vi "openCamera.vi"(0 "error in":errorcluster, 2 "Camera Settings":T2={"Camera"=enum."left_hand_camera", "FPS"=20.0, "Camera Controls"=[{"id"=0, "value"=0}, {"id"=101, "value"=-1}, {"id"=102, "value"=-1}, {"id"=103, "value"=-1}, {"id"=104, "value"=-1}, {"id"=105, "value"=-1}, {"id"=106, "value"=-1}, {"id"=107, "value"=-1}, {"id"=108, "value"=-1}, {"id"=109, "value"=1}], "Resolution"=enum."(320, 200)"}, 3 "node":string) -> (1 "error out":errorcluster)   [LabVIEW 2012]
doc: "Opens a connection to a Baxter Camera"
uses:
  ROS/Code/SubVIs/_ROSDirection.ctl
  ROS/Code/Console/Servers/ServerSubs/TopicDef.ctl
  ROS/Code/SubVIs/BaxterCamera.ctl
panel:
  out "Reply":string
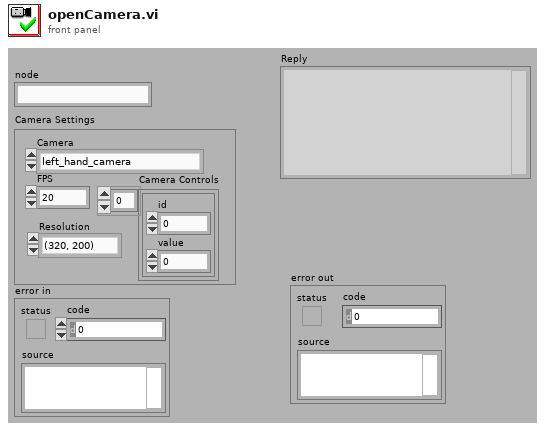
[diagram p1: front panel]
types:
  T1 = typedef "BaxterCamera.ctl" = enum16{"left_hand_camera", "right_hand_camera", "head_camera"}
  T2 = cluster{"Camera":T1, "FPS":sgl, "Camera Controls":cluster{"id":i32, "value":i32}[], "Resolution":enum16{"(1280, 800)", "(960, 600)", "(640, 400)", "(480, 300)", "(384, 240)", "(320, 200)"}}
  T3 = typedef "TopicDef.ctl" = cluster{"Topic":string, "Type":string, "Action":T4, "Update (ms)":u16, "queue size":u16}
  T4 = typedef "_ROSDirection.ctl" = enum16{"Node", "Publisher", "Subscriber", "ServiceClient", "ServiceProvider"}
  T5 = enum16{"(1280, 800)", "(960, 600)", "(640, 400)", "(480, 300)", "(384, 240)", "(320, 200)"}
  T6 = typedef "_ROSControl.ctl" = cluster{"topic port":u16, "Node":string, "topic":string, "type":string, "node port":u16, "error ":errorcluster, "Direction":T4, "Update (ms)":u16, "FIFO size":u16}
  T7 = cluster{string, "FPS":sgl, "Camera Controls":cluster{"id":i32, "value":i32}[], "Resolution":enum16{"(1280, 800)", "(960, 600)", "(640, 400)", "(480, 300)", "(384, 240)", "(320, 200)"}}
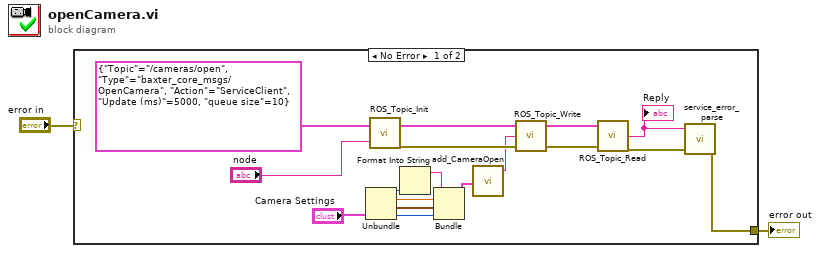
[diagram p0: block diagram]
diagram:
  n1 = case shown="No Error" "error in" {
    selector: "error in" -> [_ w20]
    tunnel: [w5 w20] -> w2
    frame No Error {
      n2 = Unbundle("Camera Settings") -> ("Camera"=w11:T1, "FPS"=w12:sgl, "Camera Controls"=w13:cluster{"id":i32, "value":i32}[], "Resolution"=w14:T5)
      n3 = call "ROS_Topic_Init.vi"("node"="node", "Definitions"=T3 {"Topic"="/cameras/open", "Type"="baxter_core_msgs/OpenCamera", "Action"=enum."ServiceClient", "Update (ms)"=5000, "queue size"=10}) -> ("error out"=w8:errorcluster, "ROS out"=w18:T6)
      n4 = Format Into String(w11) -> (resulting string=w10:string)  [unwired: 3 in, 1 out]
      n5 = Bundle(w10, "FPS"=w12, "Camera Controls"=w13, "Resolution"=w14) -> (w9:T7)  [unwired: 1 in]
      n6 = call "add_CameraOpen.vi"("Camera Settings"=w9) -> ("msg out"=w7:string)  [unwired: 4 in]
      n7 = call "ROS_Topic_Write.vi"("error in (no error)"=w8, "Msg in"=w7, "ROS in"=w18) -> ("error out"=w4:errorcluster, "ROS out"=w3:T6)  [unwired: 1 in]
      n8 = call "ROS_Topic_Read.vi"("error in (no error)"=w4, "ROS in"=w3) -> ("error out"=w6:errorcluster, "Reply"=w16:string)  [unwired: 1 in, 1 out]
      "Reply" <- w16
      n9 = call "service_error_parse.vi"("error in (no error)"=w6, "Reply"=w16) -> ("error out"=w5:errorcluster)  [unwired: 1 in, 2 out]
    }
    frame Error {
    }
  }
  "error out" <- w2
